vi "수정키보드조정읽기2.vi"() -> ()   [LabVIEW 2014]
panel:
  in  "정지":bool
  out "스페이스바3":string
  out "스페이스바  2":string
  out "스페이스바":string
  out "S":string
  out "A":string
  out "D":string
  out "W":string
  out "로컬변수":i16[](array[numeric])
  out "숫자형":i32
  out "가로":i32
  out "세로":i32
  out "키의 코드값":i16[](array[numeric])
  in  "stop 2":bool
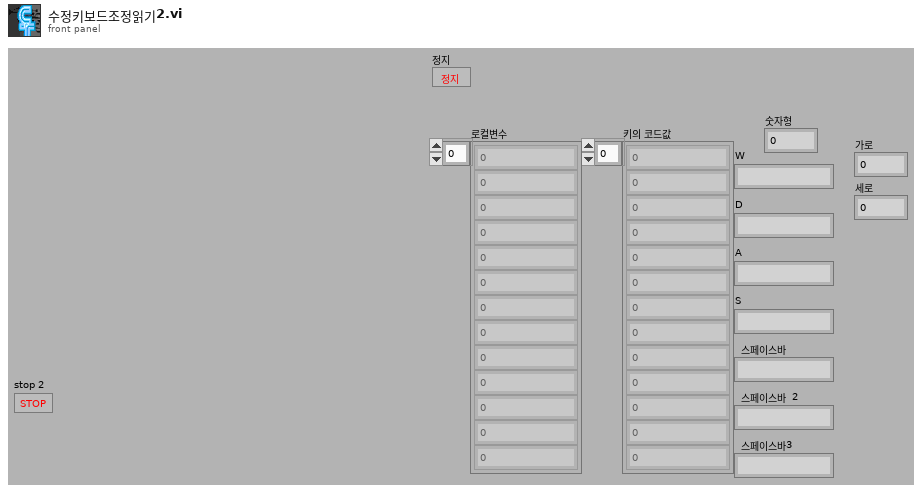
[diagram p1: front panel]
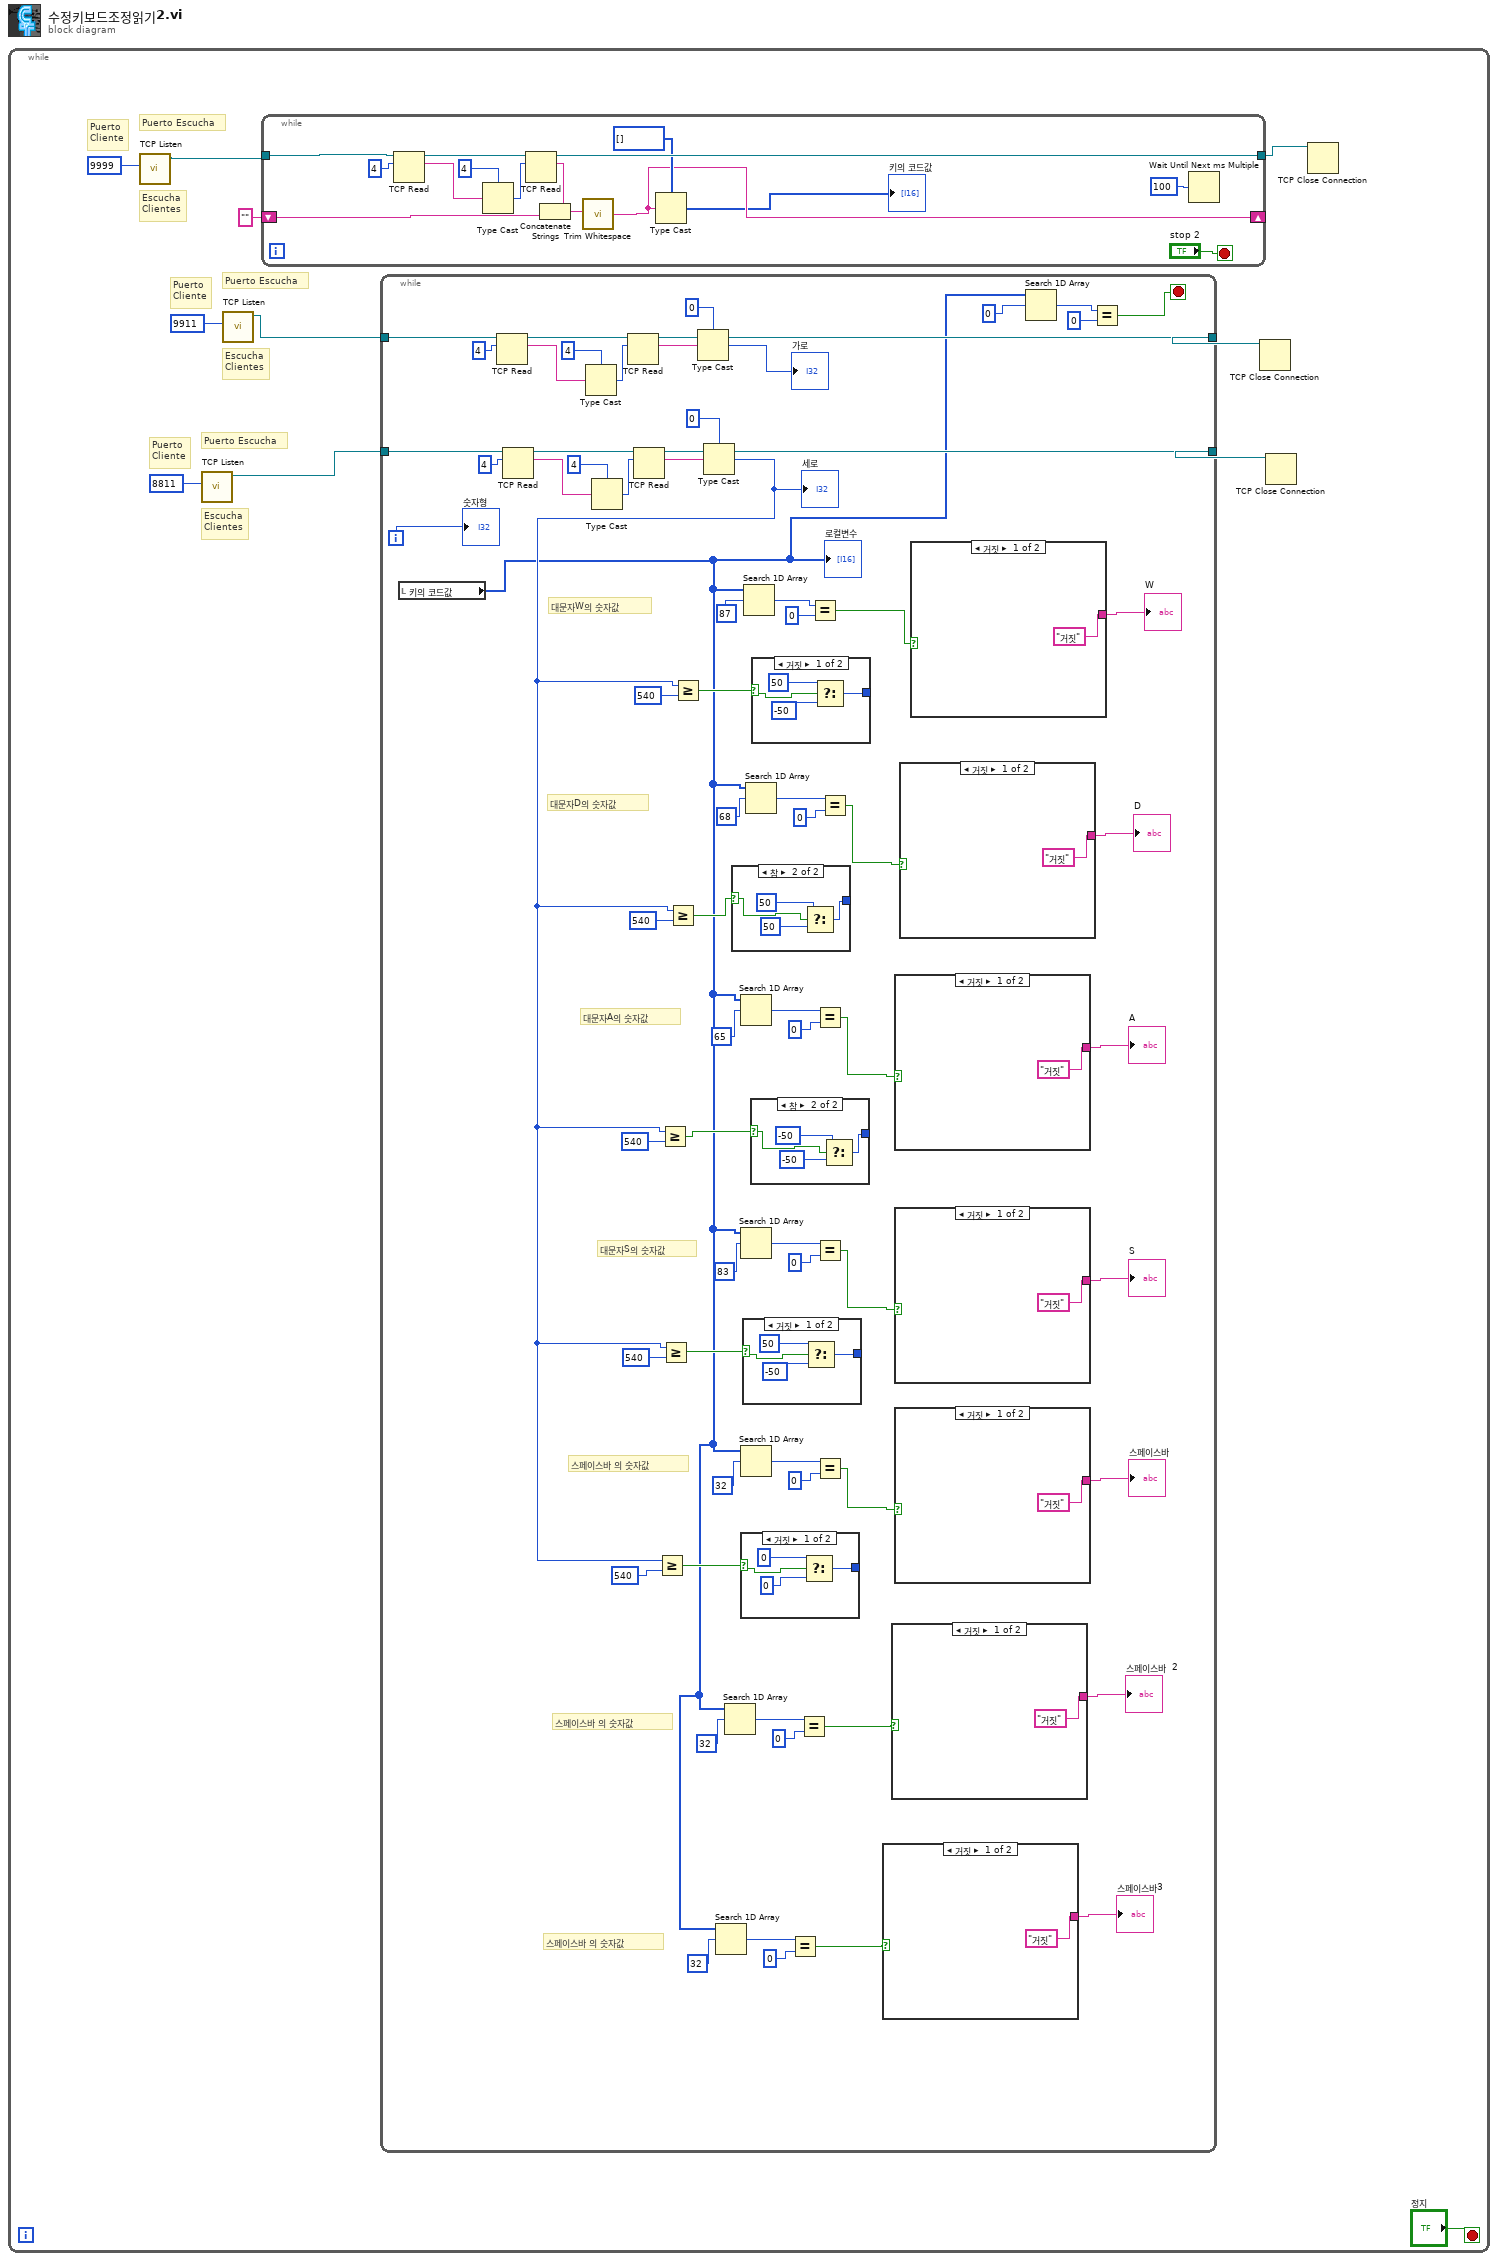
[diagram p0: block diagram]
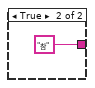
[diagram p2: hidden frame]
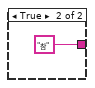
[diagram p3: hidden frame]
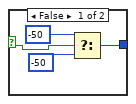
[diagram p4: hidden frame]
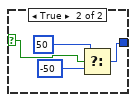
[diagram p5: hidden frame]
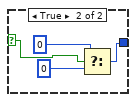
[diagram p6: hidden frame]
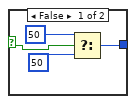
[diagram p7: hidden frame]
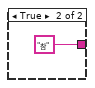
[diagram p8: hidden frame]
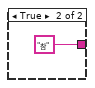
[diagram p9: hidden frame]
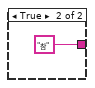
[diagram p10: hidden frame]
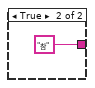
[diagram p11: hidden frame]
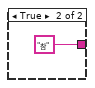
[diagram p12: hidden frame]
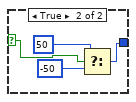
[diagram p13: hidden frame]
diagram:
  n1 = while {
    stop <- "정지" stop-if-true
    # "Puerto\nCliente"
    # "Escucha\nClientes"
    # "Puerto Escucha"
    # "Puerto\nCliente"
    # "Escucha\nClientes"
    # "Puerto Escucha"
    # "Puerto\nCliente"
    # "Escucha\nClientes"
    # "Puerto Escucha"
    n2 = call <vilib>:"TCP Listen.vi"("port"=u16 9999) -> ("connection ID"=w6:refnum<k5>)  [unwired: 6 in, 4 out]
    n3 = call <vilib>:"TCP Listen.vi"("port"=u16 8811) -> ("connection ID"=w3:refnum<k5>)  [unwired: 6 in, 4 out]
    n4 = call <vilib>:"TCP Listen.vi"("port"=u16 9911) -> ("connection ID"=w2:refnum<k5>)  [unwired: 6 in, 4 out]
    n5 = while {
      tunnel: w6 -> [w140]
      tunnel: [w150] -> w11
      shift-right: [w138] -> _
      shift-left: "" -> [w143]
      stop <- "stop 2" stop-if-true
      n6 = TCP Read(connection ID=w140, bytes to read=4) -> (connection ID out=w146:refnum<k5>, data out=w148:string)  [unwired: 3 in, 1 out]
      n7 = Type Cast(type=4 ("bytes to read"), x=w148) -> (*(type *) &x=w145:i32)
      n8 = TCP Read(connection ID=w146, bytes to read=w145) -> (connection ID out=w150:refnum<k5>, data out=w142:string)  [unwired: 3 in, 1 out]
      n9 = Concatenate Strings(w142, w143) -> (w139:string)
      n10 = call <vilib>:"Trim Whitespace.vi"("string"=w139) -> ("trimmed string"=w138:string)  [unwired: 1 in]
      n11 = Type Cast(type=i16[] [], x=w138) -> (*(type *) &x=→"키의 코드값":i16[])
      n12 = Wait Until Next ms Multiple(millisecond multiple=u32 100) -> ()  [unwired: 1 out]
    }
    n13 = while {
      tunnel: w2 -> [w82]
      tunnel: [w80] -> w9
      tunnel: w3 -> [w67]
      tunnel: [w69] -> w8
      i -> [w32]
      stop <- w34 stop-if-true
      # "스페이스바 의 숫자값"
      # "스페이스바 의 숫자값"
      # "대문자W의 숫자값"
      # "대문자D의 숫자값"
      # "대문자A의 숫자값"
      # "대문자S의 숫자값"
      # "스페이스바 의 숫자값"
      n14 = local read "키의 코드값"() -> (w12:i16[])
      "로컬변수" <- w12
      n15 = TCP Read(connection ID=w82, bytes to read=4) -> (connection ID out=w81:refnum<k5>, data out=w77:string)  [unwired: 3 in, 1 out]
      n16 = TCP Read(connection ID=w67, bytes to read=4) -> (connection ID out=w68:refnum<k5>, data out=w72:string)  [unwired: 3 in, 1 out]
      n17 = Type Cast(type=4 ("bytes to read"), x=w77) -> (*(type *) &x=w76:i32)
      n18 = Type Cast(type=4 ("bytes to read"), x=w72) -> (*(type *) &x=w73:i32)
      n19 = TCP Read(connection ID=w81, bytes to read=w76) -> (connection ID out=w80:refnum<k5>, data out=w75:string)  [unwired: 3 in, 1 out]
      n20 = TCP Read(connection ID=w68, bytes to read=w73) -> (connection ID out=w69:refnum<k5>, data out=w74:string)  [unwired: 3 in, 1 out]
      n21 = Type Cast(type=0, x=w75) -> (*(type *) &x=→"가로":i32)
      n22 = Type Cast(type=0, x=w74) -> (*(type *) &x=w23:i32)
      "세로" <- w23
      n23 = Greater Or Equal?(x=w23, y=540) -> (x >= y?=w28:bool)
      n24 = Greater Or Equal?(x=w23, y=540) -> (x >= y?=w24:bool)
      n25 = Greater Or Equal?(x=w23, y=540) -> (x >= y?=w26:bool)
      n26 = Greater Or Equal?(x=w23, y=540) -> (x >= y?=w30:bool)
      n27 = Greater Or Equal?(x=w23, y=540) -> (x >= y?=w63:bool)
      n28 = Search 1D Array(1D array=w12, element=i16 32 ("원소")) -> (index of element=w15:i32)  [unwired: 1 in]
      n29 = Search 1D Array(1D array=w12, element=i16 32 ("원소")) -> (index of element=w20:i32)  [unwired: 1 in]
      n30 = case shown="참" w30 {
        selector: w30 -> [w114 w115]
        tunnel: [w111 w116] -> _
        frame False {
          n31 = Select(t=50, s=w114, f=50) -> (s? t:f=w111:i32)
        }
        frame True {
          n32 = Select(t=50, s=w115, f=50) -> (s? t:f=w116:i32)
        }
      }
      n33 = Search 1D Array(1D array=w12, element=i16 65 ("원소")) -> (index of element=w49:i32)  [unwired: 1 in]
      n34 = Search 1D Array(1D array=w12, element=i16 83 ("원소")) -> (index of element=w48:i32)  [unwired: 1 in]
      n35 = Search 1D Array(1D array=w12, element=i16 32 ("원소")) -> (index of element=w41:i32)  [unwired: 1 in]
      n36 = case shown="거짓" w28 {
        selector: w28 -> [w106 w107]
        tunnel: [w103 w108] -> _
        frame False {
          n37 = Select(t=0, s=w106, f=0) -> (s? t:f=w103:i32)
        }
        frame True {
          n38 = Select(t=0, s=w107, f=0) -> (s? t:f=w108:i32)
        }
      }
      n39 = case shown="거짓" w26 {
        selector: w26 -> [w98 w99]
        tunnel: [w95 w100] -> _
        frame False {
          n40 = Select(t=50, s=w98, f=-50) -> (s? t:f=w95:i32)
        }
        frame True {
          n41 = Select(t=50, s=w99, f=-50) -> (s? t:f=w100:i32)
        }
      }
      n42 = Search 1D Array(1D array=w12, element=i16 87 ("원소")) -> (index of element=w59:i32)  [unwired: 1 in]
      n43 = Search 1D Array(1D array=w12, element=i16 68 ("원소")) -> (index of element=w57:i32)  [unwired: 1 in]
      n44 = case shown="참" w24 {
        selector: w24 -> [w90 w91]
        tunnel: [w87 w92] -> _
        frame False {
          n45 = Select(t=-50, s=w90, f=-50) -> (s? t:f=w87:i32)
        }
        frame True {
          n46 = Select(t=-50, s=w91, f=-50) -> (s? t:f=w92:i32)
        }
      }
      n47 = case shown="거짓" w63 {
        selector: w63 -> [w132 w133]
        tunnel: [w129 w134] -> _
        frame False {
          n48 = Select(t=50, s=w132, f=-50) -> (s? t:f=w129:i32)
        }
        frame True {
          n49 = Select(t=50, s=w133, f=-50) -> (s? t:f=w134:i32)
        }
      }
      n50 = Equal?(x=w15, y=0) -> (x = y?=w17:bool)
      n51 = Equal?(x=w20, y=0) -> (x = y?=w18:bool)
      n52 = Equal?(x=w59, y=0) -> (x = y?=w56:bool)
      n53 = Equal?(x=w49, y=0) -> (x = y?=w51:bool)
      n54 = Equal?(x=w48, y=0) -> (x = y?=w46:bool)
      n55 = Equal?(x=w41, y=0) -> (x = y?=w43:bool)
      n56 = Equal?(x=w57, y=0) -> (x = y?=w54:bool)
      n57 = case shown="거짓" w17 {
        tunnel: ["거짓" "참"] -> w13
        frame False {
        }
        frame True {
        }
      }
      "스페이스바3" <- w13
      n58 = case shown="거짓" w18 {
        tunnel: ["거짓" "참"] -> w22
        frame False {
        }
        frame True {
        }
      }
      "스페이스바  2" <- w22
      n59 = case shown="거짓" w51 {
        tunnel: ["거짓" "참"] -> w50
        frame False {
        }
        frame True {
        }
      }
      "A" <- w50
      n60 = case shown="거짓" w46 {
        tunnel: ["거짓" "참"] -> w47
        frame False {
        }
        frame True {
        }
      }
      "S" <- w47
      n61 = case shown="거짓" w43 {
        tunnel: ["거짓" "참"] -> w42
        frame False {
        }
        frame True {
        }
      }
      "스페이스바" <- w42
      n62 = case shown="거짓" w54 {
        tunnel: ["거짓" "참"] -> w55
        frame False {
        }
        frame True {
        }
      }
      "D" <- w55
      n63 = case shown="거짓" w56 {
        tunnel: ["거짓" "참"] -> w61
        frame False {
        }
        frame True {
        }
      }
      "W" <- w61
      n64 = Search 1D Array(1D array=w12, element=i16 0 ("원소")) -> (index of element=w36:i32)  [unwired: 1 in]
      n65 = Equal?(x=w36, y=0) -> (x = y?=w34:bool)
      "숫자형" <- w32
    }
    n66 = TCP Close Connection(connection ID=w9) -> ()  [unwired: 2 in, 2 out]
    n67 = TCP Close Connection(connection ID=w8) -> ()  [unwired: 2 in, 2 out]
    n68 = TCP Close Connection(connection ID=w11) -> ()  [unwired: 2 in, 2 out]
  }
